vi "Start Deploy.vi"(11 "RTTarget in":refnum<class "RTTarget.lvclass">) -> (3 "RTTarget out":refnum<class "RTTarget.lvclass">)   [LabVIEW 2020, in "NI_TargetHelper.lvlib" / "RTTarget.lvclass"]
uses:
  <vilib>/TargetSupport/NI_TargetHelper/RTTarget/RTTarget.lvclass
  <vilib>/TargetSupport/NI_TargetHelper/RTTarget/RTTarget.lvclass/RTTarget.ctl
  <vilib>/TargetSupport/NI_TargetHelper/NI_TargetHelper.lvlib
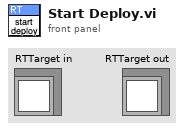
[diagram p1: front panel]
types:
  T1 = typedef "NI_TargetHelper.lvlib/Instance VIref.ctl" = refnum<vi>
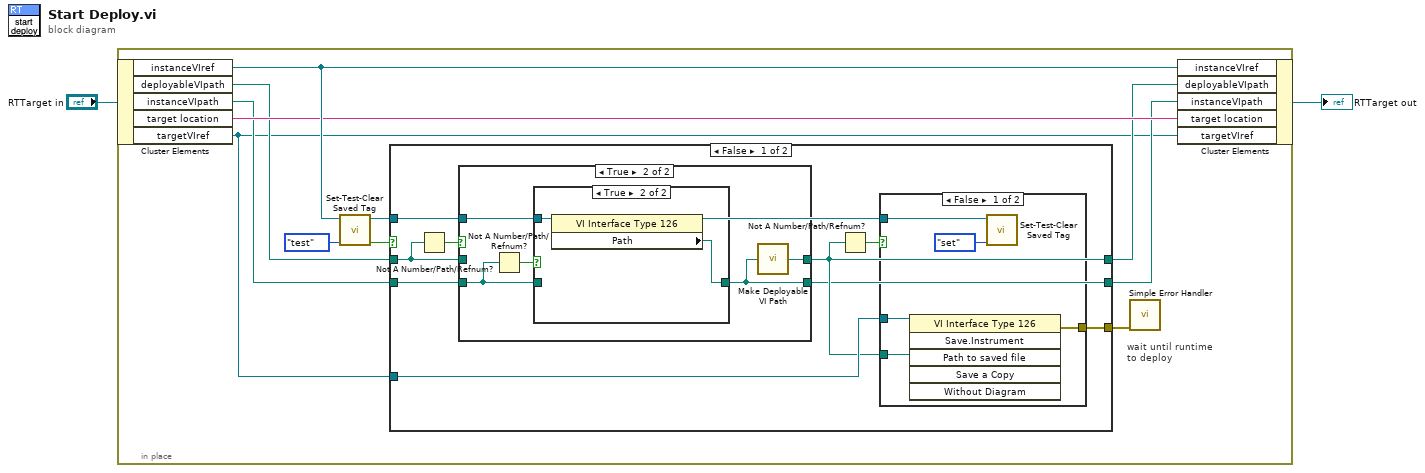
[diagram p0: block diagram]
diagram:
  n1 = in-place {
    # "wait until runtime\nto deploy"
    n2 = in-place-cluster #1("RTTarget in") -> ("instanceVIref"=w13:T1, "deployableVIpath"=w8:path, "instanceVIpath"=w5:path, "target location"=w9:string, "targetVIref"=w3:T1)
    n3 = call <vilib>:"Set-Test-Clear Saved Tag.vi"("op"=enum16{"test", "clear", "set"}."test", "instVIref"=w13) -> ("saved"=w10:bool, "instVIref out"=w12:T1)  [unwired: 8 in]
    n4 = case shown="False" w10 {
      tunnel: w12 -> [w15 _]
      tunnel: w3 -> [w18 _]
      tunnel: w5 -> [w21 w38]
      tunnel: w8 -> [w20 w39]
      tunnel: [w17 w39] -> w7
      tunnel: [w16 _] -> w6
      tunnel: [w14 w38] -> w4
      frame False {
        n5 = Not A Number/Path/Refnum?(number/path/refnum=w20) -> (NaN/Path/Refnum?=w22:bool)
        n6 = case shown="True" w22 {
          tunnel: w21 -> [w28 w31]
          tunnel: w20 -> [w29 _]
          tunnel: [w29 w34] -> w17
          tunnel: w15 -> [_ w32]
          tunnel: [w28 w30] -> w14
          frame False {
          }
          frame True {
            n7 = Not A Number/Path/Refnum?(number/path/refnum=w31) -> (NaN/Path/Refnum?=w33:bool)
            n8 = case shown="True" w33 {
              tunnel: w32 -> [_ w37]
              tunnel: [w35 w36] -> w30
              tunnel: w31 -> [w35 _]
              frame False {
              }
              frame True {
                n9 = property class="VI Interface Type 126"(reference=w37) -> ("Path"=w36:path)  [unwired: 1 in, 2 out]
              }
            }
            n10 = call <vilib>:"Make Deployable VI Path.vi"("instance path"=w30) -> ("deployable path"=w34:path)
          }
        }
        n11 = Not A Number/Path/Refnum?(number/path/refnum=w17) -> (NaN/Path/Refnum?=w19:bool)
        n12 = case shown="False" w19 {
          tunnel: w18 -> [w27 _]
          tunnel: w17 -> [w26 _]
          tunnel: w15 -> [w24 _]
          tunnel: [w23 _] -> w16
          frame False {
            n13 = invoke class="VI Interface Type 126" method="Save.Instrument"(reference=w27, "Path to saved file"=w26) -> (error out=w23:errorcluster)  [unwired: 4 in, 5 out]
            n14 = call <vilib>:"Set-Test-Clear Saved Tag.vi"("op"=enum16{"test", "clear", "set"}."set", "instVIref"=w24) -> ()  [unwired: 8 in, 2 out]
          }
          frame True {
          }
        }
      }
      frame True {
      }
    }
    n15 = call <vilib>:"Simple Error Handler.vi"("error in (no error)"=w6) -> ()  [unwired: 4 in, 5 out]
    n16 = in-place-cluster #1("instanceVIref"=w13, "deployableVIpath"=w7, "instanceVIpath"=w4, "target location"=w9, "targetVIref"=w3) -> (→"RTTarget out":refnum<class "RTTarget.lvclass">)
  }
